vi "Actor Core.vi"(8 "error in":errorcluster, 11 "State in":refnum<class "Command States.lvclass">) -> (0 "error out":errorcluster, 3 "Actor out":refnum<class "Actor.lvclass">)   [LabVIEW 2013, in "Command Actor.lvlib" / "Command States.lvclass"]
doc: "(<B>Filename</B>: Actor Framework.lvlib:Actor.lvclass:Actor Core.vi)\n\nThis override invokes Entry.vi on the initial state, prior to calling the parent Actor Core. Adding this behavior to Actor Core (instead of an override of Pre Launch Init.vi) allows the initial state to launch a nested actor as part of its entry behavior.\n\nReceives messages to the actor, reacts to them, and initiates any error handling that may shut the actor down.\n\nDescendant classes may override this VI to append parallel tasks for the actor to complete while it handles messages. Overrides use the Call Parent Method node."
uses:
  Command States.lvclass
  <vilib>/ActorFramework/Actor/Actor.lvclass
  Command/State Status.ctl
  Command States.lvclass/Command States.ctl
  <vilib>/ni/Actors/State Actor/State Actor/State Actor.lvclass
panel:
  in  "Previous State Status":T1
  in  "Current State Status":T1
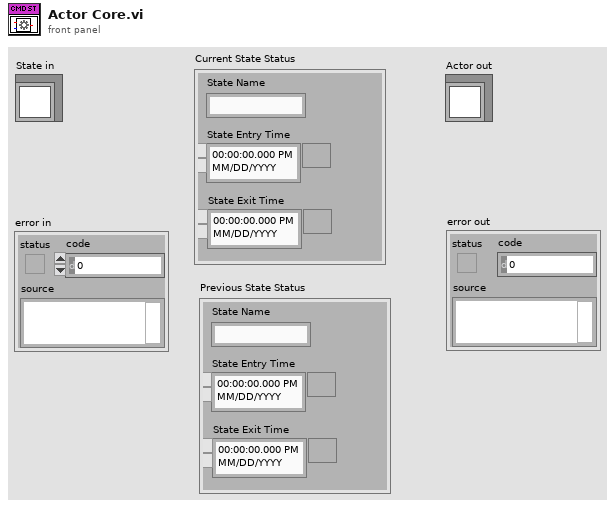
[diagram p1: front panel]
types:
  T1 = typedef "Command Actor.lvlib/Command States.lvclass/State Status.ctl" = cluster{"State Name":string, "State Entry Time":timestamp, "State Exit Time":timestamp}
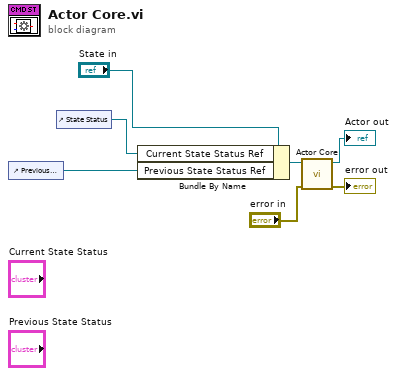
[diagram p0: block diagram]
diagram:
  n1 = control-ref of="Previous State Status"() -> (w1:refnum<vi>)
  n2 = control-ref of="State Status"() -> (w2:refnum<vi>)
  n3 = Bundle By Name(cluster="State in", "Current State Status Ref"=w2, "Previous State Status Ref"=w1) -> (w3:refnum<class "Command States.lvclass">)
  n4 = call-parent "Actor Core.vi"("error in"="error in", "State in"=w3) -> ("error out"=→"error out":errorcluster, "Actor out"=→"Actor out":refnum<class "Actor.lvclass">)  [unwired: 8 in]
